vi "1st order Filter-HP.vi"(4 "Filter Time Constant":dbl, 6 "Dt":dbl, 8 "error in":errorcluster, 11 "Data in":dbl) -> (0 "error out":errorcluster, 3 "HP data":dbl)   [LabVIEW 2014]
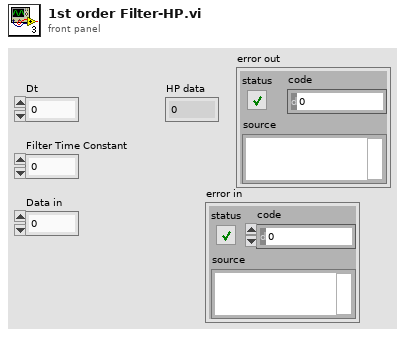
[diagram p1: front panel]
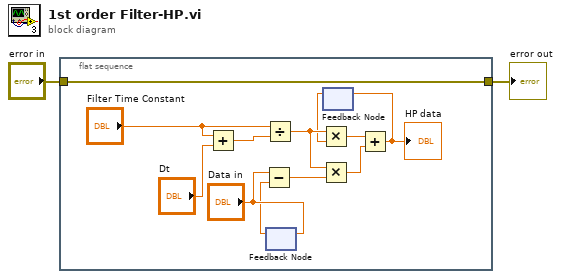
[diagram p0: block diagram]
diagram:
  n1 = flat-sequence {
    tunnel: "error in" -> [w3]
    tunnel: [w3] -> w1
    frame #0 {
      n2 = Add(x="Filter Time Constant", y="Dt") -> (x+y=w6:dbl)
      n3 = Divide(x="Filter Time Constant", y=w6) -> (x/y=w9:dbl)
      n4 = feedback #1() -> (w11:dbl)  [unwired: 1 in]
      n5 = Subtract(x="Data in", y=w11) -> (x-y=w10:dbl)
      n6 = feedback-in #1("Data in") -> ()
      n7 = Multiply(x=w9, y=w10) -> (x*y=w12:dbl)
      n8 = feedback #2() -> (w7:dbl)  [unwired: 1 in]
      n9 = Multiply(x=w9, y=w7) -> (x*y=w8:dbl)
      n10 = Add(x=w8, y=w12) -> (x+y=w13:dbl)
      "HP data" <- w13
      n11 = feedback-in #2(w13) -> ()
    }
  }
  "error out" <- w1
